vi "Facade 1.vi"(0 "Data In":T4, 2 "Display State In":T2, 3 "Container State":T3) -> (6 "Data Out":T4, 7 "Display State Out":T2, 8 "Action":T1)   [LabVIEW 2021, in "XControl 1.xctl"]
uses:
  XControl 1.xctl
  Data 1.ctl
  <vilib>/_xctls/Container State.ctl
  State 1.ctl
  <vilib>/_xctls/Action.ctl
  <vilib>/Utility/file.llb/Write Delimited Spreadsheet (string).vi
  <vilib>/_xctls/XControlSupport.lvlib
panel:
  in  "電磁閥on路徑":path=path "C:/Users/acain/Videos/專題/電磁閥/電磁閥.png"
  in  "電磁閥off路徑":path=path "C:/Users/acain/Videos/專題/電磁閥/電磁閥off.png"
  in  "常開常閉設定":bool
  in  "log存檔路徑 格式限定CSV":path=path "C:/Users/acain/Videos/專題/0726/電磁閥/電磁閥紀錄.csv"
  in  "電源開關":bool
  out "2D Picture":picture
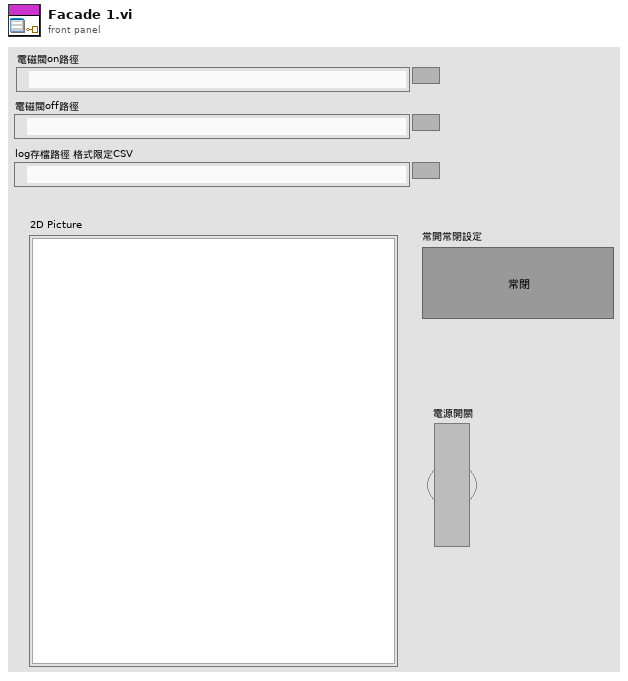
[diagram p1: front panel]
types:
  T1 = typedef "XControlSupport.lvlib/Action.ctl" = cluster{"Data Changed?":bool, "State Changed?":bool, "Action Name":string}
  T2 = typedef "XControl 1.xctl/State 1.ctl" = cluster{"Numeric":dbl}
  T3 = typedef "XControlSupport.lvlib/Container State.ctl" = cluster{"Indicator?":bool, "Run Mode?":bool, " Refnum":refnum<vi>}
  T4 = typedef "XControl 1.xctl/Data 1.ctl" = bool
  T5 = typedef "imagedata.ctl" = cluster{"image type":i32, "image depth":i32, "image":u8[], "mask":u8[], "colors":u32[], "Rectangle":cluster{"left":i16, "top":i16, "right":i16, "bottom":i16}}
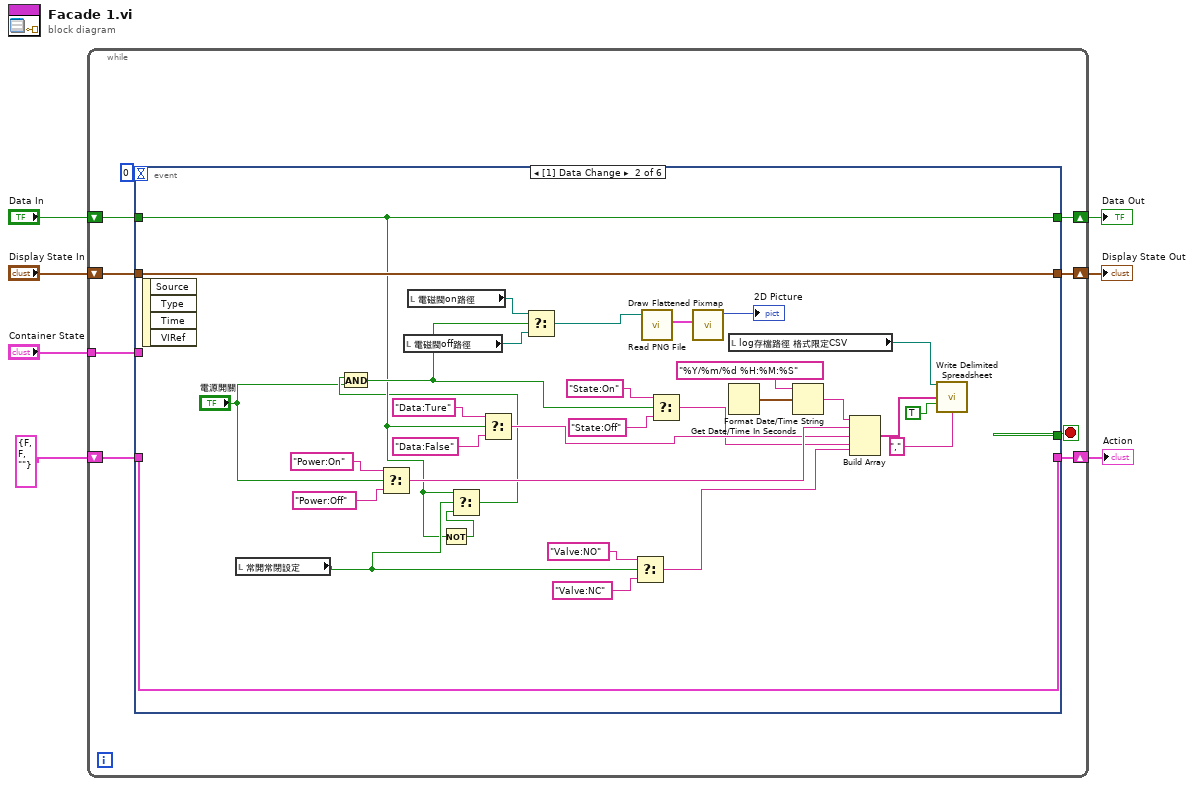
[diagram p0: block diagram]
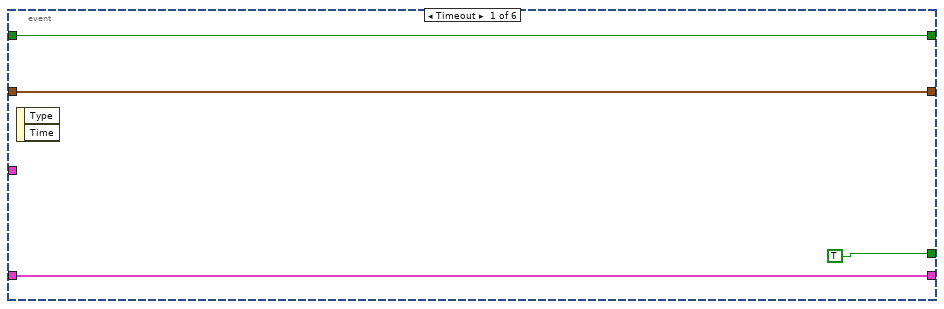
[diagram p2: hidden frame]
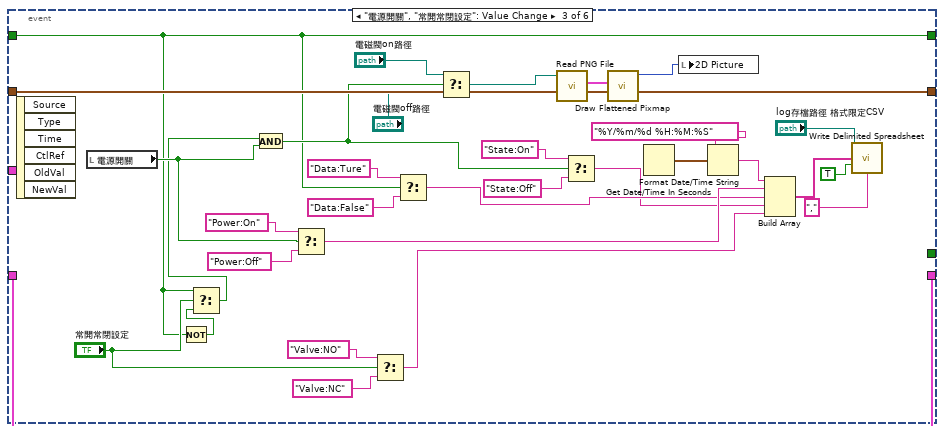
[diagram p3: hidden frame]
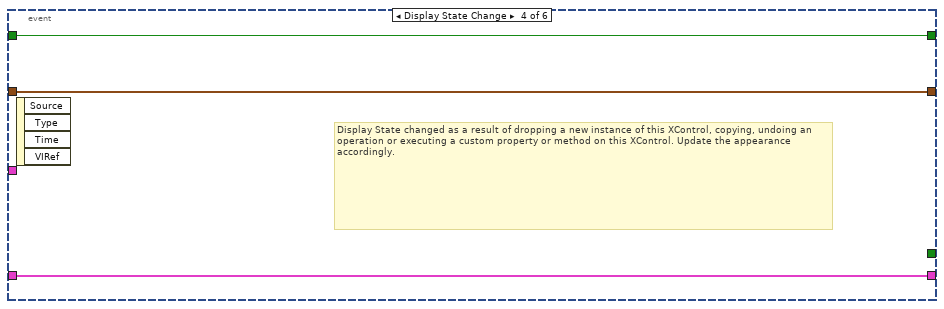
[diagram p4: hidden frame]
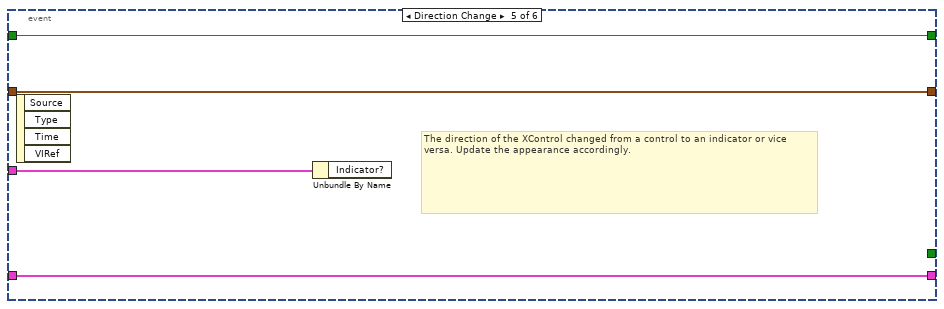
[diagram p5: hidden frame]
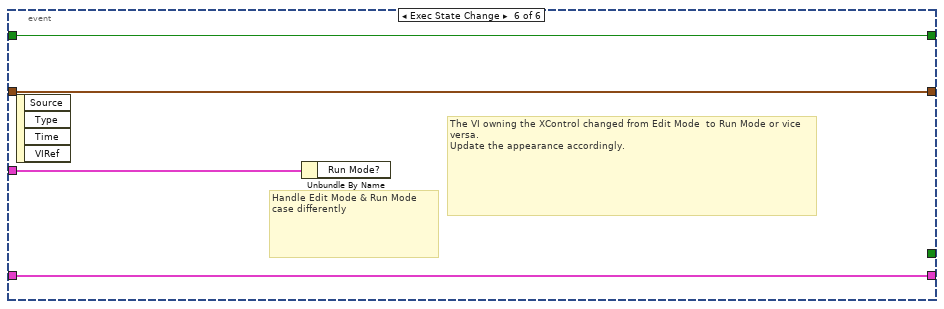
[diagram p6: hidden frame]
diagram:
  n1 = while {
    shift-right: [w15] -> w4
    shift-left: "Display State In" -> [w16]
    tunnel: "Container State" -> [w12]
    shift-right: [w10] -> w7
    shift-left: "Data In" -> [w11]
    shift-right: [w8] -> w2
    shift-left: T1 {"Data Changed?"=FALSE, "State Changed?"=FALSE, "Action Name"=""} ("Action") -> [w9]
    stop <- w14 stop-if-true
    n2 = event shown="[1] Data Change" {
      selector: _ -> [_ _ _ _ _ _]
      dyn-events: _ -> [_ _ _ _ _ _]
      timeout: 0 -> [_ _ _ _ _ _]
      tunnel: w16 -> [w18 w49 w84 w87 w90 w94]
      tunnel: [w18 w49 w84 w87 w90 w94] -> w15
      tunnel: [TRUE _ _ _ _ _] -> w14
      tunnel: w12 -> [_ _ _ _ w91 w95]
      tunnel: w11 -> [w17 w26 w55 w86 w89 w93]
      tunnel: [w17 w26 w55 w86 w89 w93] -> w10
      tunnel: [w19 w37 w83 w85 w88 w92] -> w8
      tunnel: w9 -> [w19 w37 w83 w85 w88 w92]
      event Timeout {
        n3 = event-data() -> ()  [unwired: 1 in, 2 out]
      }
      event Data Change {
        n4 = event-data() -> ()  [unwired: 1 in, 4 out]
        n5 = local read "常開常閉設定"() -> (w27:bool)
        n6 = Select(t="Power:On" ("time format string (%c)"), s="電源開關", f="Power:Off" ("time format string (%c)")) -> (s? t:f=w34:string)
        n7 = local read "電磁閥off路徑"() -> (w22:path)
        n8 = local read "電磁閥on路徑"() -> (w21:path)
        n9 = Not(x=w26) -> (.not. x?=w28:T4)
        n10 = Select(t=w26, s=w27, f=w28) -> (s? t:f=w25:T4)
        n11 = And(x=w25, y="電源開關") -> (x .and. y?=w46:T4)
        n12 = Select(t="Data:Ture" ("time format string (%c)"), s=w26, f="Data:False" ("time format string (%c)")) -> (s? t:f=w33:string)
        n13 = Select(t=w21, s=w46, f=w22) -> (s? t:f=w50:path)
        n14 = Select(t="Valve:NO" ("time format string (%c)"), s=w27, f="Valve:NC" ("time format string (%c)")) -> (s? t:f=w24:string)
        n15 = call <vilib>:"Read PNG File.vi"("path to PNG file"=w50) -> ("image data"=w52:T5)  [unwired: 8 in, 2 out]
        n16 = Select(t="State:On" ("time format string (%c)"), s=w46, f="State:Off" ("time format string (%c)")) -> (s? t:f=w32:string)
        n17 = call <vilib>:"Draw Flattened Pixmap.vi"("image data"=w52) -> ("new picture"=→"2D Picture":picture)  [unwired: 8 in]
        n18 = local read "log存檔路徑 格式限定CSV"() -> (w31:path)
        n19 = Get Date/Time In Seconds() -> (seconds since 1Jan1904=w48:timestamp)
        n20 = Format Date/Time String(time format string (%c)="%Y/%m/%d %H:%M:%S", seconds (now)=w48) -> (date/time string=w43:string)  [unwired: 1 in]
        n21 = Build Array(w43, w34, w33, w32, w24) -> (w41:string[])
        n22 = call-poly <vilib>:"Write Delimited Spreadsheet.vi"("file path (dialog if empty)"=w31, "1D data"=w41, "append to file? (new file:F)"=TRUE, "delimiter (\\t)"="," ("delimiter (\\t)")) -> ()  [unwired: 10 in, 2 out]
      }
      event "電源開關", "常開常閉設定": Value Change {
        n23 = event-data() -> ()  [unwired: 1 in, 6 out]
        n24 = local read "電源開關"() -> (w59:bool)
        n25 = Not(x=w55) -> (.not. x?=w57:T4)
        n26 = Select(t=w55, s="常開常閉設定", f=w57) -> (s? t:f=w54:T4)
        n27 = And(x=w54, y=w59) -> (x .and. y?=w79:T4)
        n28 = Select(t="Power:On" ("time format string (%c)"), s=w59, f="Power:Off" ("time format string (%c)")) -> (s? t:f=w76:string)
        n29 = Select(t="Valve:NO" ("time format string (%c)"), s="常開常閉設定", f="Valve:NC" ("time format string (%c)")) -> (s? t:f=w53:string)
        n30 = Select(t="Data:Ture" ("time format string (%c)"), s=w55, f="Data:False" ("time format string (%c)")) -> (s? t:f=w75:string)
        n31 = Select(t="電磁閥on路徑", s=w79, f="電磁閥off路徑") -> (s? t:f=w81:path)
        n32 = call <vilib>:"Read PNG File.vi"("path to PNG file"=w81) -> ("image data"=w82:T5)  [unwired: 8 in, 2 out]
        n33 = Select(t="State:On" ("time format string (%c)"), s=w79, f="State:Off" ("time format string (%c)")) -> (s? t:f=w74:string)
        n34 = call <vilib>:"Draw Flattened Pixmap.vi"("image data"=w82) -> ("new picture"=w62:picture)  [unwired: 8 in]
        n35 = Get Date/Time In Seconds() -> (seconds since 1Jan1904=w80:timestamp)
        n36 = local write "2D Picture"(w62) -> ()
        n37 = Format Date/Time String(time format string (%c)="%Y/%m/%d %H:%M:%S", seconds (now)=w80) -> (date/time string=w78:string)  [unwired: 1 in]
        n38 = Build Array(w78, w76, w75, w74, w53) -> (w77:string[])
        n39 = call-poly <vilib>:"Write Delimited Spreadsheet.vi"("file path (dialog if empty)"="log存檔路徑 格式限定CSV", "1D data"=w77, "append to file? (new file:F)"=TRUE, "delimiter (\\t)"="," ("delimiter (\\t)")) -> ()  [unwired: 10 in, 2 out]
      }
      event Display State Change {
        # "Display State changed as a result of dropping a new instance of this XControl, copying, undoing an operation or executing a custom property or method on this XControl. Update the appearance accordingly."
        n40 = event-data() -> ()  [unwired: 1 in, 4 out]
      }
      event Direction Change {
        # "The direction of the XControl changed from a control to an indicator or vice versa. Update the appearance accordingly."
        n41 = event-data() -> ()  [unwired: 1 in, 4 out]
        n42 = Unbundle By Name(w91) -> ()  [unwired: 1 out]
      }
      event Exec State Change {
        # "The VI owning the XControl changed from Edit Mode  to Run Mode or vice versa.\nUpdate the appearance accordingly."
        # "Handle Edit Mode & Run Mode\ncase differently"
        n43 = event-data() -> ()  [unwired: 1 in, 4 out]
        n44 = Unbundle By Name(w95) -> ()  [unwired: 1 out]
      }
    }
  }
  "Display State Out" <- w4
  "Data Out" <- w7
  "Action" <- w2
